vi "SBG_Ellipse_convert_to_little_endian (SubVI) (1).vi"(4 "string":string) -> (1 "String":string)   [LabVIEW 2017]
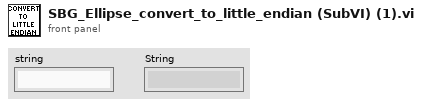
[diagram p1: front panel]
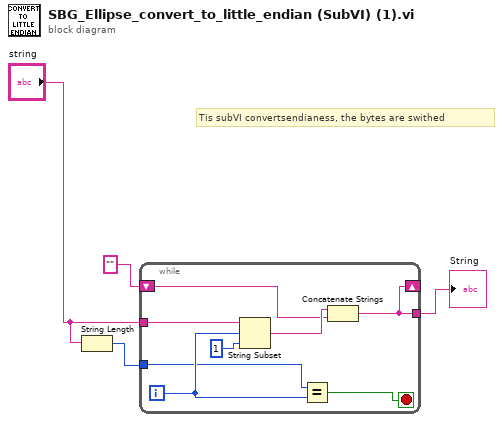
[diagram p0: block diagram]
diagram:
  # "Tis subVI convertsendianess, the bytes are swithed"
  n1 = String Length(string="string") -> (length=w2:i32)
  n2 = while {
    tunnel: "string" -> [w11]
    tunnel: [w7] -> w1
    tunnel: w2 -> [w8]
    shift-right: [w7] -> _
    shift-left: "" -> [w5]
    i -> [w9]
    stop <- w10 stop-if-true
    n3 = String Subset(string=w11, offset (0)=w9, length (rest)=1 ("length (rest)")) -> (substring=w6:string)
    n4 = Equal?(x=w8, y=w9) -> (x = y?=w10:bool)
    n5 = Concatenate Strings(w6, w5) -> (w7:string)
  }
  "String" <- w1
